vi "open_rga_interface.vi"() -> ()   [LabVIEW 2016]
panel:
  out "standard output":string
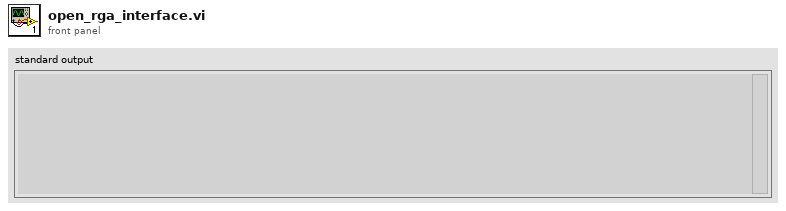
[diagram p1: front panel]
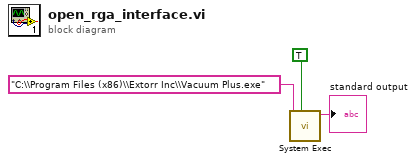
[diagram p0: block diagram]
diagram:
  n1 = call <vilib>:"System Exec.vi"("wait until completion? (T)"=TRUE, "command line"="C:\\Program Files (x86)\\Extorr Inc\\Vacuum Plus.exe") -> ("standard output"=→"standard output":string)  [unwired: 6 in, 3 out]
